vi "Search in Array.vi"(5 "items to filter":string[](array[string]), 6 "array":string[](array[string])) -> (1 "item Indexs":i32[](array[numeric]), 2 "array(dup)":string[](array[string]))   [LabVIEW 2017, in "TagDB RefManager.lvlib"]
doc: "This polymorphic VI filters out all instances of <B>items to filter</B> from the input <B>array</B> and outputs the result as <B>filtered array</B> along with an array of <B>filtered item indices</B> containing the indices of the items that were filtered. You can wire either a 1D array or a scalar value to <B>items to filter</B>."
uses:
  TagDB RefManager.lvlib
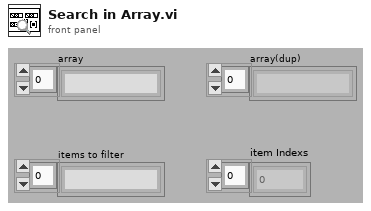
[diagram p1: front panel]
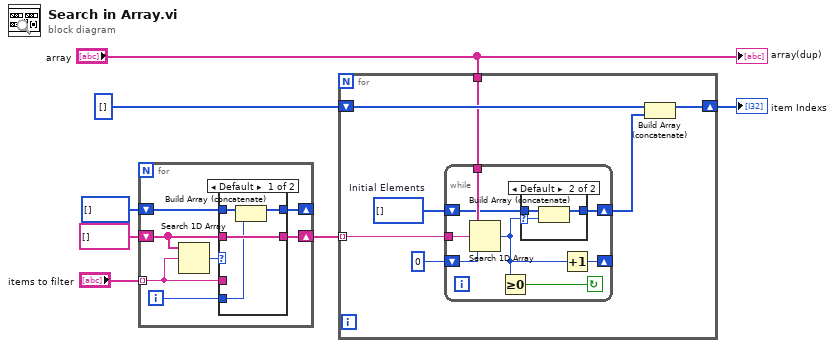
[diagram p0: block diagram]
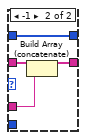
[diagram p3: hidden frame]
diagram:
  n1 = for {
    tunnel: "items to filter" -> [w13] mode=indexing
    shift-right: [w12] -> w3
    shift-left: string[] [] -> [w11]
    shift-right: [w9] -> _
    shift-left: i32[] [] -> [w8]
    i -> [w10]
    n2 = Search 1D Array(1D array=w11, element=w13) -> (index of element=w14:i32)  [unwired: 1 in]
    n3 = case shown="Default" w14 {
      tunnel: w13 -> [_ w22]
      tunnel: [w18 w20] -> w12
      tunnel: w11 -> [w18 w21]
      tunnel: w10 -> [w15 _]
      tunnel: [w16 w19] -> w9
      tunnel: w8 -> [w17 w19]
      frame Default {
        n4 = Build Array (concatenate)(w17, w15) -> (w16:i32[])
      }
      frame -1 {
        n5 = Build Array (concatenate)(w21, w22) -> (w20:string[])
      }
    }
  }
  n6 = for {
    tunnel: w3 -> [w29] mode=indexing
    shift-right: [w27] -> w4
    shift-left: i32[] [] -> [w26]
    tunnel: "array" -> [w25]
    w23 = i32[] []  # Initial Elements
    n7 = while {
      shift-right: [w30] -> _
      shift-left: 0 ("Start Index (0)") -> [w37]
      shift-right: [w34] -> w28
      shift-left: w23 -> [w35]
      tunnel: w25 -> [w36]
      tunnel: w29 -> [w33]
      stop <- w31 continue-if-true
      n8 = Search 1D Array(1D array=w36, element=w33, start index (0)=w37) -> (index of element=w32:i32)
      n9 = Greater Or Equal To 0?(x=w32) -> (x >= 0?=w31:bool)
      n10 = case shown="Default" w32 {
        selector: w32 -> [_ w41]
        tunnel: w35 -> [w38 w40]
        tunnel: [w38 w39] -> w34
        frame -1 {
        }
        frame Default {
          n11 = Build Array (concatenate)(w40, w41) -> (w39:i32[])
        }
      }
      n12 = Increment(x=w32) -> (x+1=w30:i32)
    }
    n13 = Build Array (concatenate)(w26, w28) -> (w27:i32[])
  }
  "item Indexs" <- w4
  "array(dup)" <- "array"
